vi "Read sequence info from MAT file.vi"(8 "error in":errorcluster, 11 "Movie file name":path) -> (0 "error out":errorcluster, 1 "Description Info":string, 2 "Number of frames":u32, 3 "Header file data":T1 {"Pixel depth" items=["8 bits", "16 bits", "Float", "Complex", "RGB", "HSL"]; "time of 1st frame, \nsec since 1/1/04" format="%.2f"})   [LabVIEW 2011]
doc: "Writes a documentation file (in Matlabs MAT format) to accompany an AVI or stacked-TIFF movie. The only contents of the file will be a structure named 'vid'. Read the file using the Matlab 'load' command:\n\n>> load 16.01.mat\n>> vid\n\nvid = \n\n moviefile: '\\\\Jg_i\\c-drive\\LabView development\\Glimpse\\junk4\\16.01.tif'\n username: 'gelles'\n description: 'GLIMPSE v. 36 (8/04)'\n nframes: 5\n time1: 3.1555e+009\n ttb: [300 334 367 400 434]\n depth: 0\n\nNotes on the elements of the structure:\n\nnframes -- number of frames in the movie\ntime1 -- time of acquisition of the first frame in seconds from Jan 1, 1904\nttb -- timestamps of frames in milliseconds\ndepth -- 0 <-> 8-bit; 1 <-> 16-bit"
uses:
  Header file data.ctl
  Seq file v 1/Offset table.ctl
  Seq file v 1/Offset.ctl
  Seq file v 1/file number.ctl
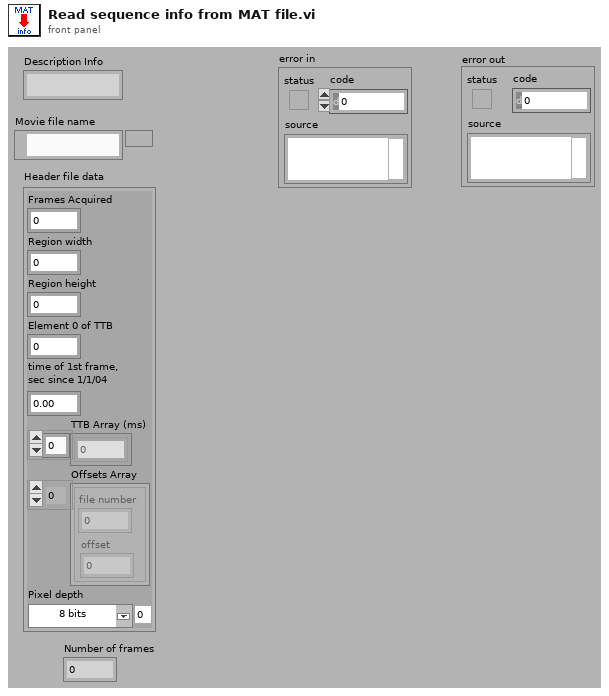
[diagram p1: front panel]
types:
  T1 = typedef "Header file data.ctl" = cluster{"Frames Acquired":u32, "Region width":i32, "Region height":i32, "Element 0 of TTB":u32, "time of 1st frame, \nsec since 1/1/04":dbl, "TTB Array (ms)":u32[], "Offsets Array":T2, "Pixel depth":u32}
  T2 = typedef "Offset table.ctl" = cluster{"offset":T3, "file number":T4}[]
  T3 = typedef "Offset.ctl" = i32
  T4 = typedef "file number.ctl" = u8
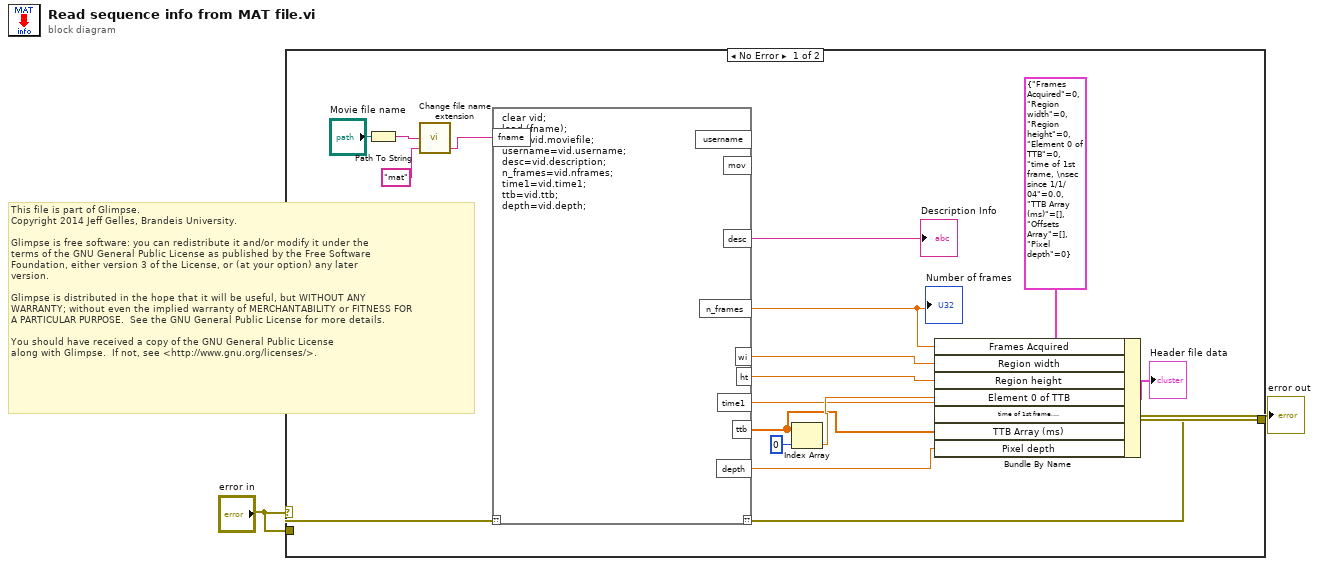
[diagram p0: block diagram]
diagram:
  # "This file is part of Glimpse. \nCopyright 2014 Jeff Gelles, Brandeis University.    \n\nGlimpse is free software: you can redistribute it and/or modify it under the \nterms of the GNU General Public License as published by the Free Software \nFoundation, either version 3 of the License, or (at your option) any later \nversion.\n\nGlimpse is distributed in the hope that it will be useful, but WITHOUT ANY \nWARRANTY; without even the implied warranty of MERCHANTABILITY or FITNESS FOR \nA PARTICULAR PURPOSE.  See the GNU General Public License for more details.\n\nYou should have received a copy of the GNU General Public License\nalong with Glimpse.  If not, see <http://www.gnu.org/licenses/>."
  n1 = case shown="No Error" "error in" {
    tunnel: "error in" -> [w17 w20]
    tunnel: [w14 w20] -> w2
    frame No Error {
      n2 = Path To String(path="Movie file name") -> (string=w3:string)
      n3 = call "Change file name extension.vi"("New Extension (no period)"="mat", "Path String In"=w3) -> ("New Path String Out"=w18:string)  [unwired: 3 out]
      n4 = script code="clear vid;\nload (fname);\nmov=vid.moviefile;\nusername=vid.username;\ndesc=vid.description;\nn_frames=vid.nframes;\ntime1=vid.time1;\nttb=vid.ttb;\ndepth=vid.depth;"("??"=w17, "fname"=w18) -> ("??"=w14:errorcluster, "n_frames"=w10:dbl, "wi"=w9:dbl, "ht"=w8:dbl, "ttb"=w6:dbl[], "depth"=w4:dbl, "time1"=w5:dbl, "desc"=→"Description Info":string)  [unwired: 2 out]
      "Number of frames" <- w10
      n5 = Index Array(array=w6, index=0) -> (element=w7:dbl)
      n6 = Bundle By Name(cluster=T1 {"Frames Acquired"=0, "Region width"=0, "Region height"=0, "Element 0 of TTB"=0, "time of 1st frame, \nsec since 1/1/04"=0.0, "TTB Array (ms)"=[], "Offsets Array"=[], "Pixel depth"=0} ("Header file data"), "Frames Acquired"=w10, "Region width"=w9, "Region height"=w8, "Element 0 of TTB"=w7, "time of 1st frame, \nsec since 1/1/04"=w5, "TTB Array (ms)"=w6, "Pixel depth"=w4) -> (→"Header file data":T1)
    }
    frame Error {
    }
  }
  "error out" <- w2
